vi "estimatedTime.vi"(10 "time (ms)":dbl, 11 "Start time":string) -> (3 "total time":dbl)   [LabVIEW 2021]
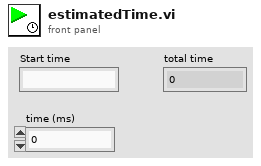
[diagram p1: front panel]
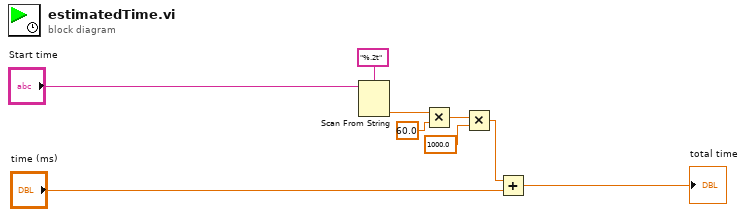
[diagram p0: block diagram]
diagram:
  n1 = Scan From String(format string="%.2t", input string="Start time") -> (output 1=w3:dbl)  [unwired: 3 in, 3 out]
  n2 = Multiply(x=w3, y=60.0) -> (x*y=w6:dbl)
  n3 = Multiply(x=w6, y=1000.0) -> (x*y=w8:dbl)
  n4 = Add(x=w8, y="time (ms)") -> (x+y=→"total time":dbl)
